vi "Destroy.vi"(0 "reference in":refnum<class "NS slave.lvclass">, 5 "error in (no error)":errorcluster) -> (14 "reference out":refnum<class "NS slave.lvclass">, 19 "error out":errorcluster)   [LabVIEW 2019, in "CommandResponse communication.lvlib" / "NS slave.lvclass"]
doc: "Destructor."
uses:
  NS slave.lvclass
  CR slave_class/CR slave.lvclass
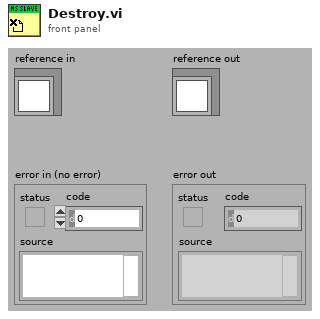
[diagram p1: front panel]
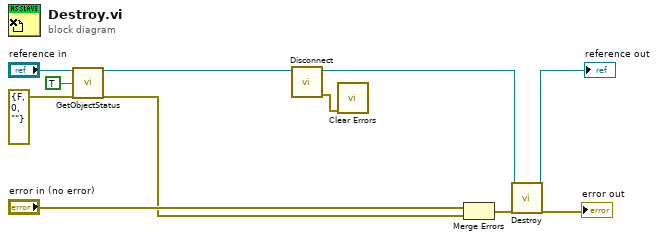
[diagram p0: block diagram]
diagram:
  n1 = call-dynamic "GetObjectStatus.vi"("reference in"="reference in", "simple info (F)"=TRUE ("simple info"), "error in (no error)"=errorcluster {"status"=FALSE, "code"=0, "source"=""}) -> ("reference out"=w3:refnum<class "NS slave.lvclass">, "error out"=w4:errorcluster)  [unwired: 5 in, 10 out]
  n2 = call-dynamic "Disconnect.vi"("reference in"=w3) -> ("error out"=w1:errorcluster, "reference out"=w2:refnum<class "NS slave.lvclass">)  [unwired: 9 in]
  n3 = call <vilib>:"Clear Errors.vi"("error in (no error)"=w1) -> ()  [unwired: 5 in, 2 out]
  n4 = Merge Errors("error in (no error)", w4) -> (w10:errorcluster)
  n5 = call-parent "Destroy.vi"("reference in"=w2, "error in (no error)"=w10) -> ("reference out"=→"reference out":refnum<class "NS slave.lvclass">, "error out"=→"error out":errorcluster)  [unwired: 16 in]
